vi "createPubDataEvents.vi"(8 "error in (no error)":errorcluster, 11 "UserEvents in":refnum<class "UserEvents.lvclass">) -> (0 "error out":errorcluster, 3 "UserEvents out":refnum<class "UserEvents.lvclass">)   [LabVIEW 2012, in "UserEvents.lvclass"]
uses:
  UserEvents.lvclass
  Typedefs/StateSelector.ctl
  Program Files (x86)/National Instruments/LabVIEW 2012/user.lib/Common/ILC/Typedefs/OutputData.ctl
  Program Files (x86)/National Instruments/LabVIEW 2012/user.lib/Common/ILC/Configuration/ILCConfig.ctl
  Program Files (x86)/National Instruments/LabVIEW 2012/user.lib/Common/ILC/Configuration/InputChannels.ctl
  Program Files (x86)/National Instruments/LabVIEW 2012/user.lib/Common/ILC/Configuration/ScanRate_Hz_MultichannelOptions.ctl
  Program Files (x86)/National Instruments/LabVIEW 2012/user.lib/Common/ILC/Typedefs/InputData.ctl
  Program Files (x86)/National Instruments/LabVIEW 2012/user.lib/Common/ILC/Typedefs/LimitSwitches.ctl
  Program Files (x86)/National Instruments/LabVIEW 2012/user.lib/Common/ILC/Typedefs/ADCs.ctl
  UserEvents.lvclass/UserEvents.ctl
  Program Files (x86)/National Instruments/LabVIEW 2012/user.lib/Common/ILC/Typedefs/ILCTypedefs.lvlib
  Program Files (x86)/National Instruments/LabVIEW 2012/user.lib/Common/ILC/Configuration/ILCConfiguration.lvlib
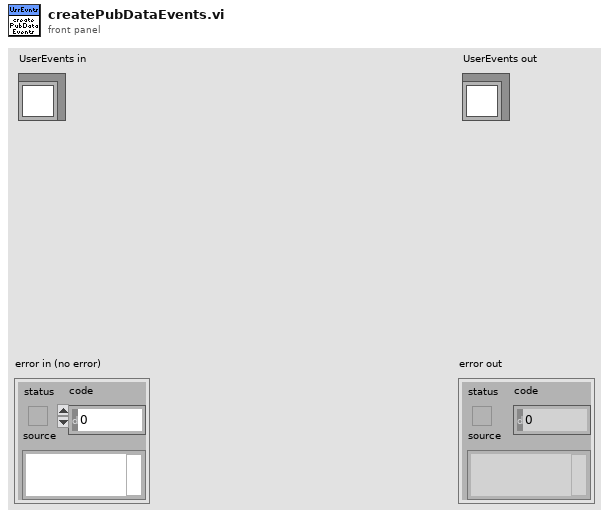
[diagram p1: front panel]
types:
  T1 = typedef "ILCCommon.lvlib/ILCTypedefs.lvlib/InputData.ctl" = cluster{"Input Channels":T2, "Limit Switches":T3, "Tachometer":u16, "SSI Encoder":i32, "ADCs":T4}
  T2 = typedef "ILCCommon.lvlib/ILCConfiguration.lvlib/InputChannels.ctl" = enum16{"Channel 0", "3 Channels", "5 Channels"}
  T3 = typedef "ILCCommon.lvlib/ILCTypedefs.lvlib/LimitSwitches.ctl" = cluster{"1":bool, "2":bool}
  T4 = typedef "ILCCommon.lvlib/ILCTypedefs.lvlib/ADCs.ctl" = cluster{"Ch1":i32, "Ch2":i32, "Ch3":i32, "Ch4":i32, "Ch5":i32}
  T5 = typedef "ILCCommon.lvlib/ILCConfiguration.lvlib/ILCConfig.ctl" = cluster{"Input Channels":T2, "Scan Rate (Hz) ":T6, "ADC PGA Gain":u8}
  T6 = typedef "ILCCommon.lvlib/ILCConfiguration.lvlib/ScanRate_Hz_MultichannelOptions.ctl" = enum16{"50", "60", "100", "120", "200", "240", "300", "400", "480", "600", "1200", "2400", "4800"}
  T7 = typedef "ILCCommon.lvlib/ILCTypedefs.lvlib/OutputData.ctl" = cluster{"Step & Direction":i16, "Blower RPM":u8, "PWM (SSR)":u8, "Ch1":u16, "Ch2":u16, "Ch3":u16, "Ch4":u16}
  T8 = typedef "StateSelector.ctl" = enum16{"DataOnDemandState", "DataStreamingState", "FaultState", "OffState", "StandbyState"}
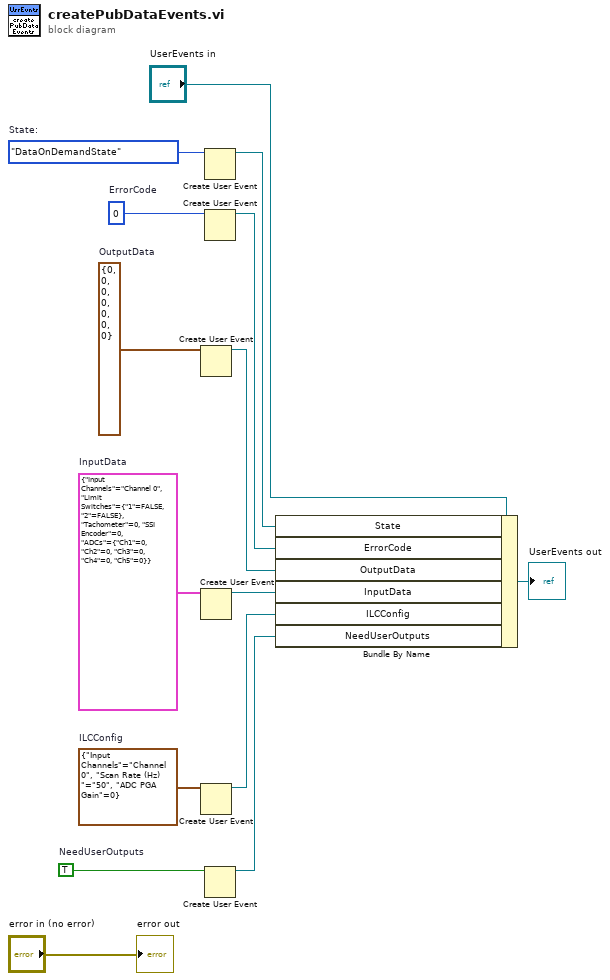
[diagram p0: block diagram]
diagram:
  w2 = TRUE  # NeedUserOutputs
  w8 = T1 {"Input Channels"=enum."Channel 0", "Limit Switches"={"1"=FALSE, "2"=FALSE}, "Tachometer"=0, "SSI Encoder"=0, "ADCs"={"Ch1"=0, "Ch2"=0, "Ch3"=0, "Ch4"=0, "Ch5"=0}}  # InputData
  w9 = T5 {"Input Channels"=enum."Channel 0", "Scan Rate (Hz) "=enum."50", "ADC PGA Gain"=0}  # ILCConfig
  w10 = T7 {"Step & Direction"=0, "Blower RPM"=0, "PWM (SSR)"=0, "Ch1"=0, "Ch2"=0, "Ch3"=0, "Ch4"=0}  # OutputData
  w11 = 0  # ErrorCode
  w12 = StateSelector."DataOnDemandState"  # State:
  n1 = Create User Event(user event datatype=w10) -> (user event=w5:refnum<user-event>)  [unwired: 1 in, 1 out]
  n2 = Create User Event(user event datatype=w8) -> (user event=w4:refnum<user-event>)  [unwired: 1 in, 1 out]
  n3 = Create User Event(user event datatype=w9) -> (user event=w3:refnum<user-event>)  [unwired: 1 in, 1 out]
  n4 = Create User Event(user event datatype=w12) -> (user event=w7:refnum<user-event>)  [unwired: 1 in, 1 out]
  n5 = Create User Event(user event datatype=w11) -> (user event=w6:refnum<user-event>)  [unwired: 1 in, 1 out]
  n6 = Create User Event(user event datatype=w2) -> (user event=w1:refnum<user-event>)  [unwired: 1 in, 1 out]
  n7 = Bundle By Name(cluster="UserEvents in", "State"=w7, "ErrorCode"=w6, "OutputData"=w5, "InputData"=w4, "ILCConfig"=w3, "NeedUserOutputs"=w1) -> (→"UserEvents out":refnum<class "UserEvents.lvclass">)
  "error out" <- "error in (no error)"
